vi "Stop Core.vi"(10 "final error code":i32, 11 "Graph in":refnum<class "Graph.lvclass">) -> (3 "Graph out":refnum<class "Graph.lvclass">)   [LabVIEW 2020, in "Graph.lvlib" / "Graph.lvclass"]
doc: "(<B>Filename</B>: Actor Framework.lvlib:Actor.lvclass:Stop Core.vi)\n\nDefines what the actor does before it stops. Use the <B>final error code</B> input to determine whether the actor shut down in response to an error.\n\nThis implementation destroys the user events and closes the chart refnum."
uses:
  Graph.lvclass
  Graph.lvclass/Graph.ctl
  PPL/HDH.Actor Framework.Core.Actor.lvlibp/1abvi3w/vi.lib/ActorFramework/Actor/Actor.lvclass
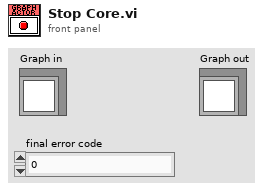
[diagram p1: front panel]
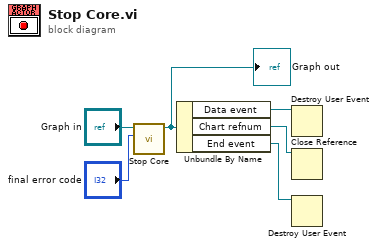
[diagram p0: block diagram]
diagram:
  n1 = call-parent "Stop Core.vi"("final error code"="final error code", "Actor in"="Graph in") -> ("Actor out"=w4:refnum<class "Graph.lvclass">)  [unwired: 9 in]
  "Graph out" <- w4
  n2 = Unbundle By Name(w4) -> ("Data event"=w3:refnum<user-event>, "Chart refnum"=w2:refnum<vi>, "End event"=w1:refnum<user-event>)
  n3 = Destroy User Event(user event=w3) -> ()  [unwired: 1 in, 1 out]
  n4 = Close Reference(reference=w2) -> ()  [unwired: 1 in, 1 out]
  n5 = Destroy User Event(user event=w1) -> ()  [unwired: 1 in, 1 out]
